vi "MarkerStyle.vi"(1 "Enum MarkerStyle":u16) -> (0 "MarkerStyle":string)   [LabVIEW 2025]
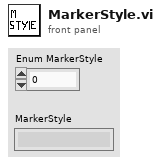
[diagram p1: front panel]
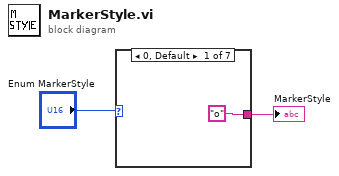
[diagram p0: block diagram]
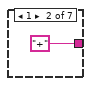
[diagram p2: hidden frame]
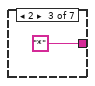
[diagram p3: hidden frame]
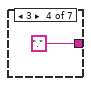
[diagram p4: hidden frame]
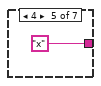
[diagram p5: hidden frame]
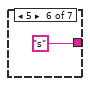
[diagram p6: hidden frame]
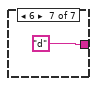
[diagram p7: hidden frame]
diagram:
  n1 = case shown="0, Default" "Enum MarkerStyle" {
    tunnel: ["o" "+" "*" "." "x" "s" "d"] -> w2
    frame 0, Default {
    }
    frame 1 {
    }
    frame 2 {
    }
    frame 3 {
    }
    frame 4 {
    }
    frame 5 {
    }
    frame 6 {
    }
  }
  "MarkerStyle" <- w2
